vi "ExtractPayload.vi"(10 "Received Message":u8[](array[numeric])) -> (0 "Checksum":u8[](array[numeric]), 1 "Payload":u8[](array[numeric]), 2 "Size":u32, 3 "Header":u8[](array[numeric]))   [LabVIEW 2014]
panel:
  out "Send Type":u32
  out "Data Type":u8[](array[numeric])
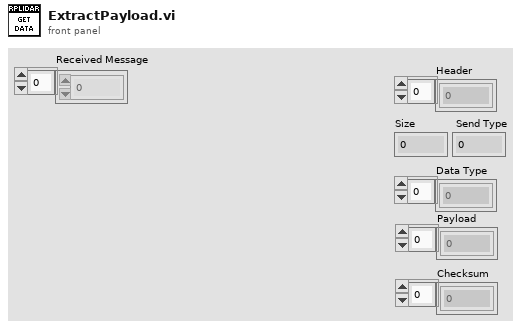
[diagram p1: front panel]
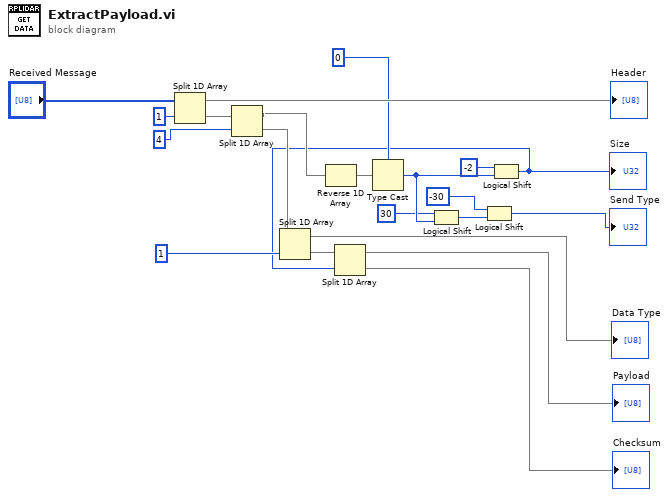
[diagram p0: block diagram]
diagram:
  n1 = Split 1D Array(array="Received Message", index=1) -> (first subarray=→"Header":u8[], second subarray=w18:u8[])
  n2 = Split 1D Array(array=w18, index=4) -> (first subarray=w11:u8[], second subarray=w16:u8[])
  n3 = Split 1D Array(array=w16, index=1) -> (first subarray=→"Data Type":u8[], second subarray=w13:u8[])
  n4 = Reverse 1D Array(array=w11) -> (reversed array=w10:u8[])
  n5 = Type Cast(type=u32 0, x=w10) -> (*(type *) &x=w7:u32)
  n6 = Logical Shift(y=30 ("x << y"), x=w7) -> (x << y=w6:u32)
  n7 = Logical Shift(y=-30 ("x << y"), x=w6) -> (x << y=→"Send Type":u32)
  n8 = Logical Shift(y=i16 -2, x=w7) -> (x << y=w1:u32)
  "Size" <- w1
  n9 = Split 1D Array(array=w13, index=w1) -> (first subarray=→"Payload":u8[], second subarray=→"Checksum":u8[])
